vi "Anheben der Amplitude (SubVi).vi"(8 "error In":errorcluster, 9 "FrequencyList Output Level (calc)":dbl=94.0, 10 "FrequencyList Input Level":dbl=94.0, 11 "custom frequency list Input":T1(array[cluster])) -> (0 "error Out":errorcluster, 1 "FrequencyList Output Level (calc)":dbl, 3 "custom frequency list Output":T1(array[cluster]))   [LabVIEW 2018]
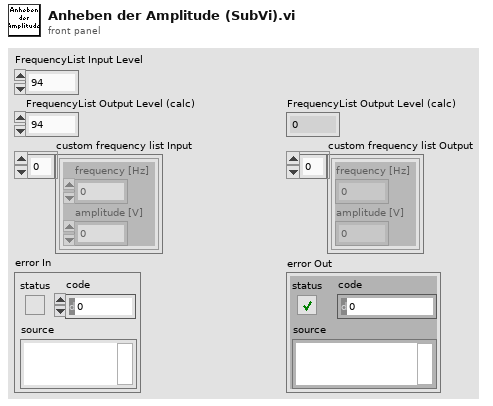
[diagram p1: front panel]
types:
  T1 = cluster{"frequency [Hz]":dbl, "amplitude [V]":dbl}[]
  T2 = cluster{"frequency [Hz]":dbl, "amplitude [V]":dbl}
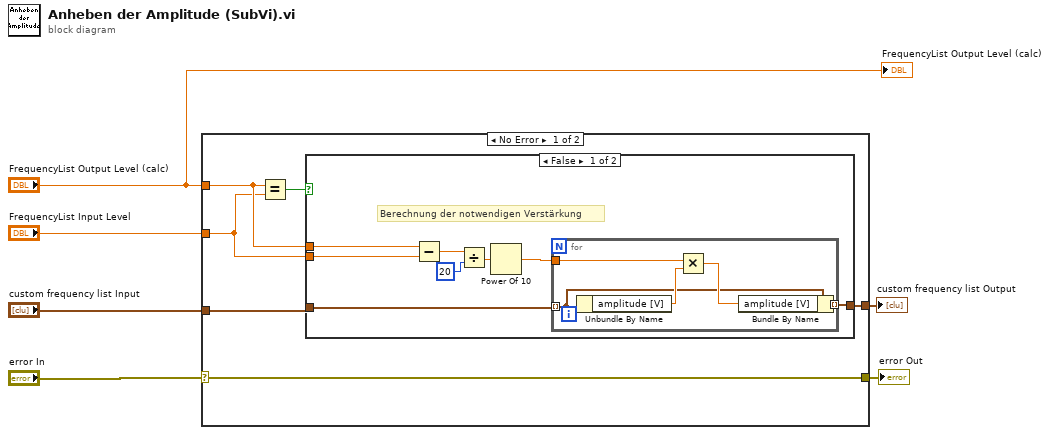
[diagram p0: block diagram]
diagram:
  n1 = case shown="No Error" "error In" {
    selector: "error In" -> [w7 w27]
    tunnel: "FrequencyList Output Level (calc)" -> [w12 _]
    tunnel: [w11 _] -> w6
    tunnel: "custom frequency list Input" -> [w10 _]
    tunnel: "FrequencyList Input Level" -> [w8 _]
    tunnel: [w7 w27] -> w2
    frame No Error {
      n2 = Equal?(x=w12, y=w8) -> (x = y?=w9:bool)
      n3 = case shown="False" w9 {
        tunnel: w10 -> [w20 w26]
        tunnel: [w19 w26] -> w11
        tunnel: w12 -> [w15 _]
        tunnel: w8 -> [w13 _]
        frame False {
          # "Berechnung der notwendigen Verstärkung"
          n4 = Subtract(x=w15, y=w13) -> (x-y=w18:dbl)
          n5 = Divide(x=w18, y=20) -> (x/y=w16:dbl)
          n6 = Power Of 10(x=w16) -> (10^x=w14:dbl)
          n7 = for {
            tunnel: w20 -> [w22] mode=indexing
            tunnel: [w25] -> w19 mode=indexing
            tunnel: w14 -> [w21]
            n8 = Unbundle By Name(w22) -> ("amplitude [V]"=w24:dbl)
            n9 = Multiply(x=w21, y=w24) -> (x*y=w23:dbl)
            n10 = Bundle By Name(cluster=w22, "amplitude [V]"=w23) -> (w25:T2)
          }
        }
        frame True {
        }
      }
    }
    frame Error {
    }
  }
  "custom frequency list Output" <- w6
  "error Out" <- w2
  "FrequencyList Output Level (calc)" <- "FrequencyList Output Level (calc)"
